vi "Get process list.vi"() -> (0 "x != y?":bool)   [LabVIEW 2010]
uses:
  kernel32.dll
  psapi.dll
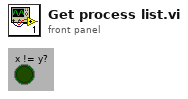
[diagram p1: front panel]
types:
  T1 = cluster{"cb":u32, "PageFaultCount":u32, "PeakWorkingSetSize":u32, "WorkingSetSize":u32, "QuotaPeakPagedPoolUsage":u32, "QuotaPagedPoolUsage":u32, "QuotaPeakNonPagedPoolUsage":u32, "QuotaNonPagedPoolUsage":u32, "PagefileUsage":u32, "PeakPagefileUsage":u32}[]
  T2 = cluster{"cb":u32, "PageFaultCount":u32, "PeakWorkingSetSize":u32, "WorkingSetSize":u32, "QuotaPeakPagedPoolUsage":u32, "QuotaPagedPoolUsage":u32, "QuotaPeakNonPagedPoolUsage":u32, "QuotaNonPagedPoolUsage":u32, "PagefileUsage":u32, "PeakPagefileUsage":u32}
  T3 = cluster{"PROCESS_MEMORY_COUNTERS":cluster{"cb":u32, "PageFaultCount":u32, "PeakWorkingSetSize":u32, "WorkingSetSize":u32, "QuotaPeakPagedPoolUsage":u32, "QuotaPagedPoolUsage":u32, "QuotaPeakNonPagedPoolUsage":u32, "QuotaNonPagedPoolUsage":u32, "PagefileUsage":u32, "PeakPagefileUsage":u32}, "ImageFileName":string}
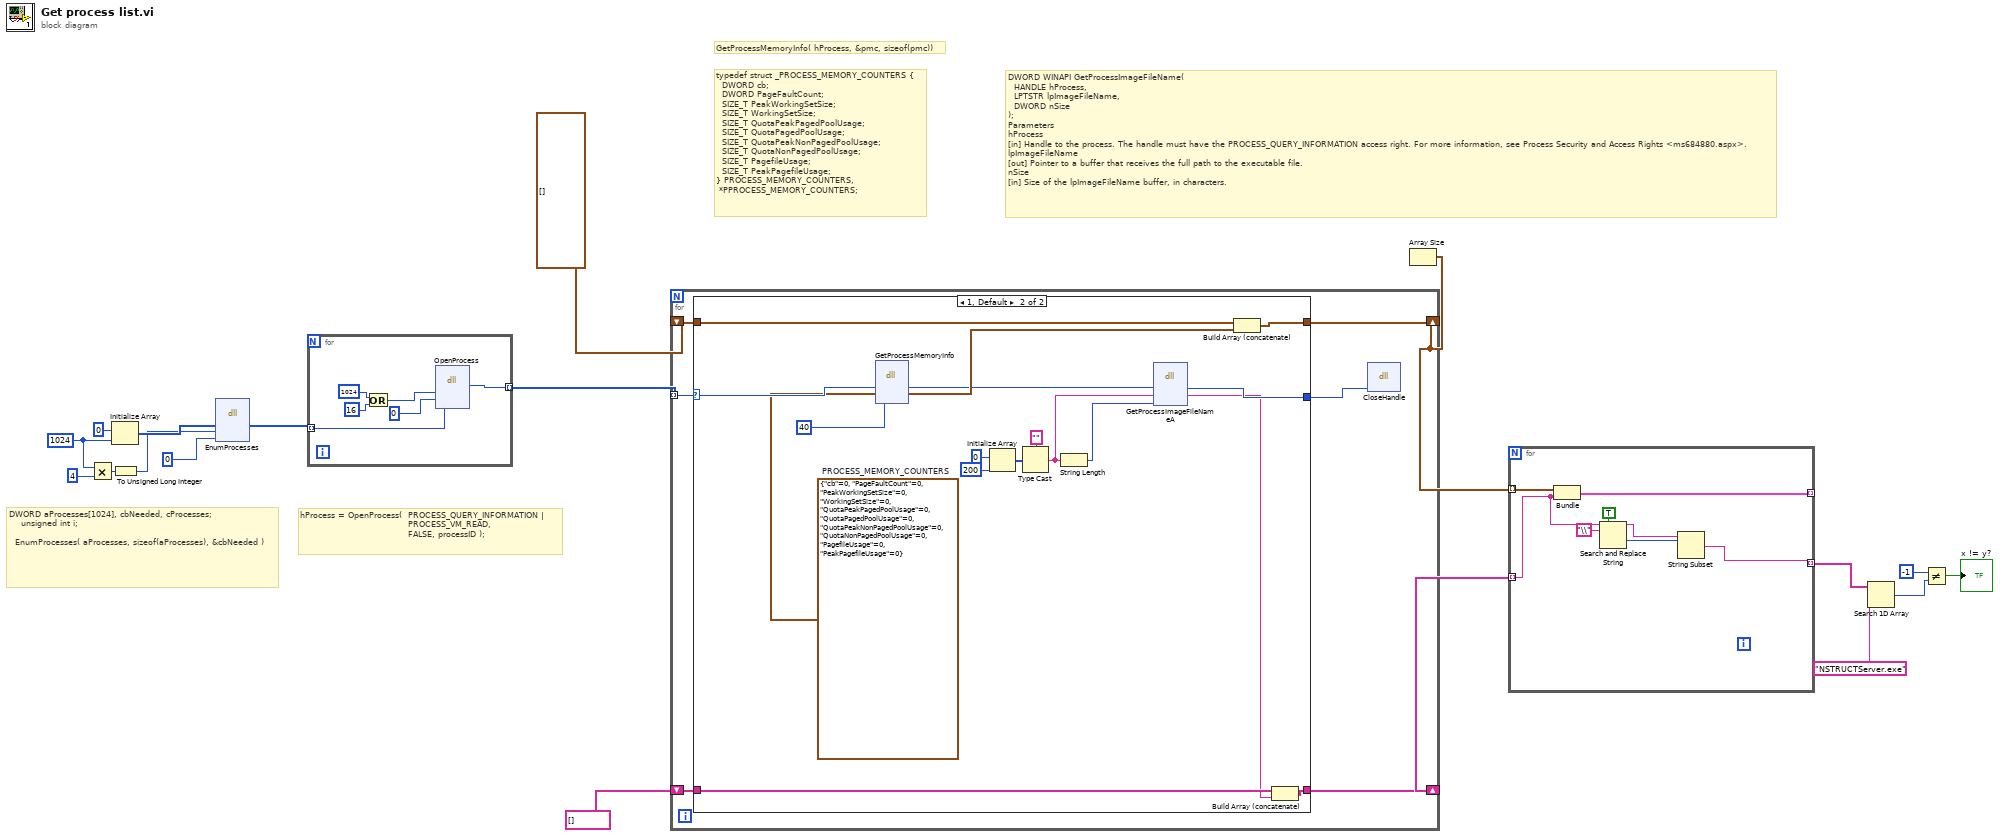
[diagram p0: block diagram]
diagram:
  w16 = u32 1024 ("dimension size")
  # "DWORD WINAPI GetProcessImageFileName(\n  HANDLE hProcess,\n  LPTSTR lpImageFileName,\n  DWORD nSize\n);\nParameters\nhProcess \n[in] Handle to the process. The handle must have the PROCESS_QUERY_INFORMATION access right. For more information, see Process Security and Access Rights <ms684880.aspx>. \nlpImageFileName \n[out] Pointer to a buffer that receives the full path to the executable file. \nnSize \n[in] Size of the lpImageFileName buffer, in characters."
  # "GetProcessMemoryInfo( hProcess, &pmc, sizeof(pmc))"
  # "typedef struct _PROCESS_MEMORY_COUNTERS {\n  DWORD cb;\n  DWORD PageFaultCount;\n  SIZE_T PeakWorkingSetSize;\n  SIZE_T WorkingSetSize;\n  SIZE_T QuotaPeakPagedPoolUsage;\n  SIZE_T QuotaPagedPoolUsage;\n  SIZE_T QuotaPeakNonPagedPoolUsage;\n  SIZE_T QuotaNonPagedPoolUsage;\n  SIZE_T PagefileUsage;\n  SIZE_T PeakPagefileUsage;\n} PROCESS_MEMORY_COUNTERS, \n *PPROCESS_MEMORY_COUNTERS;"
  # "DWORD aProcesses[1024], cbNeeded, cProcesses;\n    unsigned int i;\n\n  EnumProcesses( aProcesses, sizeof(aProcesses), &cbNeeded )"
  # "hProcess = OpenProcess(  PROCESS_QUERY_INFORMATION |\n                                    PROCESS_VM_READ,\n                                    FALSE, processID );"
  n1 = Multiply(x=w16, y=u32 4) -> (x*y=w13:u32)
  n2 = Initialize Array(u32 0 ("element"), w16) -> (w17:u32[])
  n3 = To Unsigned Long Integer(number=w13) -> (unsigned 32bit integer=w12:u32)
  n4 = dll-call lib="psapi.dll" fn="EnumProcesses"("pProcessIds"=w17, "cb"=w12, "pBytesReturned"=u32 0 ("y")) -> ("pProcessIds"=w11:u32[])  [unwired: 6 in, 2 out]
  n5 = for {
    tunnel: w11 -> [w24] mode=indexing
    tunnel: [w23] -> w9 mode=indexing
    n6 = Or(x=u32 1024 ("PROCESS_QUERY_INFORMATION"), y=u32 16 ("PROCESS_VM_READ")) -> (x .or. y?=w19:u32)
    n7 = dll-call lib="kernel32.dll" fn="OpenProcess" label="Kernel32.dll:EnumProcesses"("DesiredAccess"=w19, "InheritHandle"=0, "ProcessId"=w24) -> ("handle"=w23:i32)  [unwired: 6 in, 2 out]
  }
  n8 = for {
    tunnel: w9 -> [w30] mode=indexing
    shift-right: [w29] -> w7
    shift-left: T1 [] -> [w28]
    shift-right: [w26] -> w6
    shift-left: string[] [] -> [w25]
    n9 = case shown="1, Default" w30 {
      selector: w30 -> [w32 w50]
      tunnel: [w33 w46] -> w29
      tunnel: w28 -> [w33 w45]
      tunnel: [w32 w38] -> w27
      tunnel: [w31 w44] -> w26
      tunnel: w25 -> [w31 w43]
      frame 0 {
      }
      frame 1, Default {
        w49 = T2 {"cb"=0, "PageFaultCount"=0, "PeakWorkingSetSize"=0, "WorkingSetSize"=0, "QuotaPeakPagedPoolUsage"=0, "QuotaPagedPoolUsage"=0, "QuotaPeakNonPagedPoolUsage"=0, "QuotaNonPagedPoolUsage"=0, "PagefileUsage"=0, "PeakPagefileUsage"=0}  # PROCESS_MEMORY_COUNTERS
        n10 = dll-call lib="psapi.dll" fn="GetProcessMemoryInfo"("handle"=w50, "PROCESS_MEMORY_COUNTERS"=w49, "cb"=u32 40) -> ("handle"=w37:i32, "PROCESS_MEMORY_COUNTERS"=w47:T2)  [unwired: 5 in, 2 out]
        n11 = Initialize Array(u8 0 ("element"), 200 ("dimension size")) -> (w40:u8[])
        n12 = Type Cast(type="" ("pointerTostring"), x=w40) -> (*(type *) &x=w35:string)
        n13 = String Length(string=w35) -> (length=w36:i32)
        n14 = dll-call lib="psapi.dll" fn="GetProcessImageFileNameA" label="PSAPI.dll:GetModuleFileNameExA"("handle"=w37, "ImageFileName"=w35, "Size"=w36) -> ("handle"=w38:i32, "ImageFileName"=w34:string)  [unwired: 5 in, 2 out]
        n15 = Build Array (concatenate)(w45, w47) -> (w46:T1)
        n16 = Build Array (concatenate)(w43, w34) -> (w44:string[])
      }
    }
    n17 = dll-call lib="kernel32.dll" fn="CloseHandle" label="Kernel32.dll:EnumProcesses"("handle"=w27) -> ()  [unwired: 5 in, 2 out]
  }
  n18 = Array Size(array=w7) -> ()  [unwired: 1 out]
  n19 = for {
    tunnel: w7 -> [w57] mode=indexing
    tunnel: w6 -> [w53] mode=indexing
    tunnel: [w58] -> _ mode=indexing
    tunnel: [w51] -> w5 mode=indexing
    n20 = Bundle("PROCESS_MEMORY_COUNTERS"=w57, "ImageFileName"=w53) -> (w58:T3)  [unwired: 1 in]
    n21 = Search and Replace String(replace all?=TRUE ("replace all? (F)"), input string=w53, search string="\\") -> (result string=w52:string, offset past replacement=w54:i32)  [unwired: 5 in, 2 out]
    n22 = String Subset(string=w52, offset (0)=w54) -> (substring=w51:string)  [unwired: 1 in]
  }
  n23 = Search 1D Array(1D array=w5, element="NSTRUCTServer.exe") -> (index of element=w3:i32)  [unwired: 1 in]
  n24 = Not Equal?(x=-1, y=w3) -> (x != y?=→"x != y?":bool)
